vi "Load Becker-Hickl FLIM Data Block.vi"(4 "Compressed?":bool, 6 "Image Sizes":T1, 8 "Error In":errorcluster, 9 "Data Type":T3, 10 "Data Block Header":T2, 11 "File Path Control":path) -> (0 "Error Out":errorcluster, 2 "Data":sgl[][][](array[numeric]), 3 "File Path":path)   [LabVIEW 2021, in "Becker-Hickl Files.lvlib"]
uses:
  Becker-Hickl Files.lvlib
  Becker-Hickl Data Type.ctl
  Becker-Hickl Data Block Header.ctl
  Becker-Hickl FLIM Image Sizes.ctl
panel:
  out "Intensity Graph":sgl[][](graph)
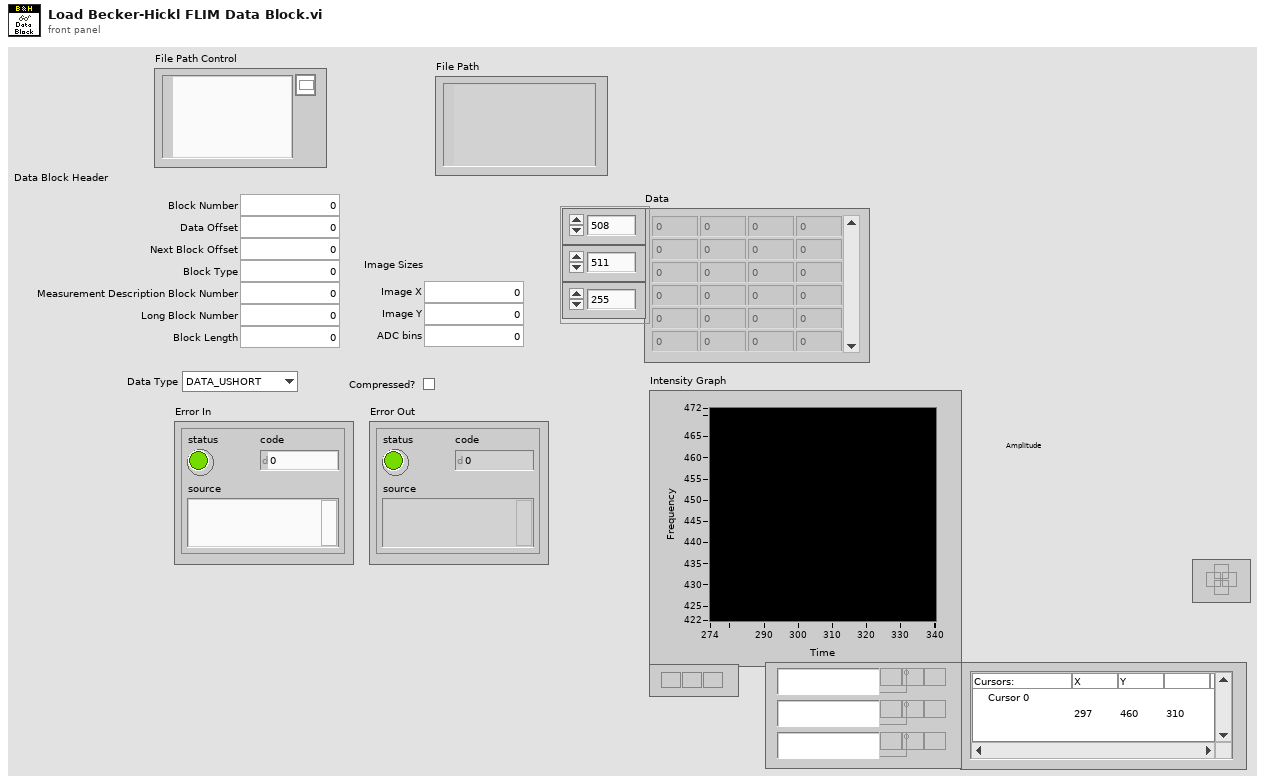
[diagram p1: front panel]
types:
  T1 = typedef "Becker-Hickl Files.lvlib/Becker-Hickl FLIM Image Sizes.ctl" = cluster{"Image X":i32, "Image Y":i32, "ADC bins":i32}
  T2 = typedef "Becker-Hickl Files.lvlib/Becker-Hickl Data Block Header.ctl" = cluster{"Block Number":u16, "Data Offset":u32, "Next Block Offset":u32, "Block Type":u16, "Measurement Description Block Number":u16, "Long Block Number":u32, "Block Length":u32}
  T3 = typedef "Becker-Hickl Files.lvlib/Becker-Hickl Data Type.ctl" = enum16{"DATA_USHORT", "DATA_ULONG", "DATA_DBL"}
  T4 = enum16{"big-endian, network order", "native, host order", "little-endian"}
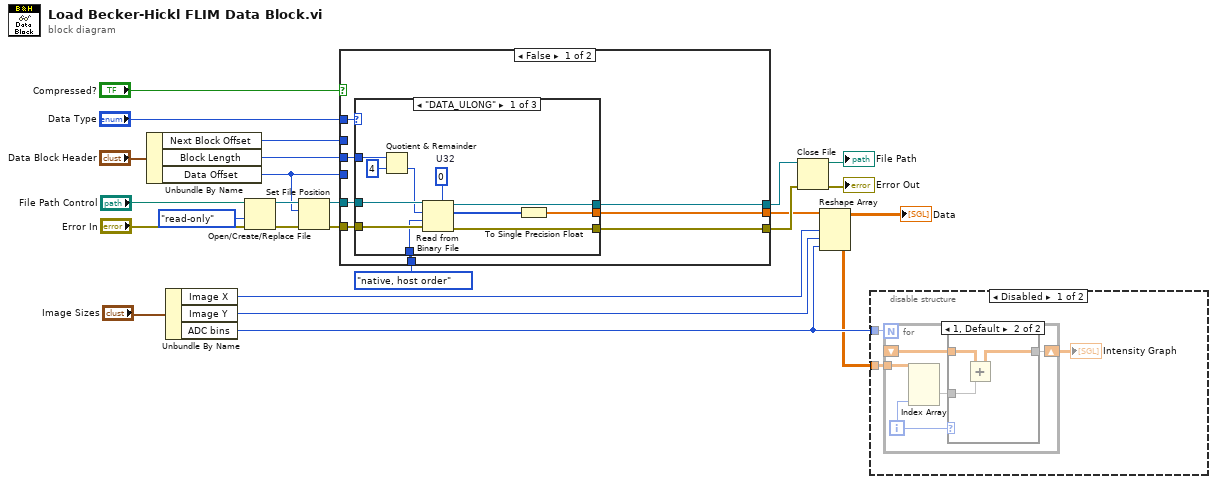
[diagram p0: block diagram]
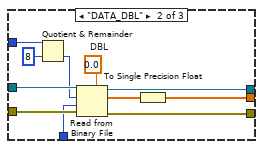
[diagram p4: hidden frame]
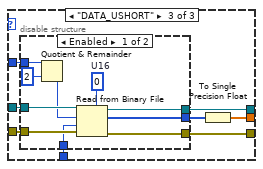
[diagram p5: hidden frame]
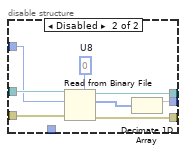
[diagram p6: hidden frame]
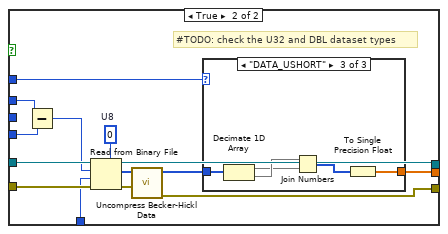
[diagram p7: hidden frame]
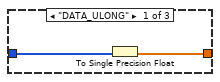
[diagram p8: hidden frame]
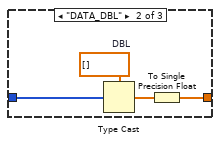
[diagram p9: hidden frame]
diagram:
  n1 = Unbundle By Name("Data Block Header") -> ("Next Block Offset"=w4:u32, "Block Length"=w15:u32, "Data Offset"=w3:u32)
  n2 = Unbundle By Name("Image Sizes") -> ("Image X"=w7:i32, "Image Y"=w6:i32, "ADC bins"=w2:i32)
  n3 = Open/Create/Replace File(file path (use dialog)="File Path Control", error in="Error In", access (0:read/write)=enum16{"read/write", "read-only", "write-only"}."read-only") -> (refnum out=w19:refnum<file>, error out=w20:errorcluster)  [unwired: 3 in, 1 out]
  n4 = Set File Position(offset (in bytes) (0)=w3, refnum=w19, error in=w20) -> (refnum out=w17:refnum<file>, error out=w16:errorcluster)  [unwired: 1 in]
  n5 = case shown="False" "Compressed?" {
    tunnel: "Data Type" -> [w32 w89]
    tunnel: w17 -> [w31 w93]
    tunnel: w16 -> [w30 w94]
    tunnel: w15 -> [w29 _]
    tunnel: [w28 w90] -> w14
    tunnel: [w27 w87] -> w13
    tunnel: [w26 w88] -> w10
    tunnel: T4."native, host order" ("byte order (0:big-endian, network order)") -> [w25 w81]
    tunnel: w4 -> [_ w92]
    tunnel: w3 -> [_ w91]
    frame False {
      n6 = case shown="\"DATA_ULONG\"" w32 {
        tunnel: w31 -> [w42 w53 w61]
        tunnel: w30 -> [w43 w54 w62]
        tunnel: w29 -> [w36 w47 w57]
        tunnel: [w40 w51 w60] -> w28
        tunnel: [w34 w45 w56] -> w26
        tunnel: [w38 w49 w58] -> w27
        tunnel: w25 -> [w33 w44 w55]
        frame "DATA_ULONG" {
          w41 = u32 0  # U32
          n7 = Quotient & Remainder(x=w36, y=u32 4) -> (floor(x/y)=w37:u32)  [unwired: 1 out]
          n8 = Read from Binary File(5:w41, 8:w43, 9:w33, 10:w37, 11:w42) -> (0:w38:errorcluster, 2:w39:u32[], 3:w40:refnum<file>)  [unwired: 1 in, 1 out]
          n9 = To Single Precision Float(number=w39) -> (single precision float=w34:sgl[])
        }
        frame "DATA_DBL" {
          w52 = 0.0  # DBL
          n10 = Quotient & Remainder(x=w47, y=u32 8) -> (floor(x/y)=w46:u32)  [unwired: 1 out]
          n11 = Read from Binary File(5:w52, 8:w54, 9:w44, 10:w46, 11:w53) -> (0:w49:errorcluster, 2:w50:dbl[], 3:w51:refnum<file>)  [unwired: 1 in, 1 out]
          n12 = To Single Precision Float(number=w50) -> (single precision float=w45:sgl[])
        }
        frame "DATA_USHORT" {
          n13 = disable-structure shown="Enabled" {
            disable-tunnel: w62 -> [w72 w80]
            disable-tunnel: w61 -> [w71 w79]
            disable-tunnel: [w69 w77] -> w60
            disable-tunnel: [w68 w73] -> w59
            disable-tunnel: [w67 w75] -> w58
            disable-tunnel: w57 -> [w65 w74]
            disable-tunnel: w55 -> [w63 _]
            frame Enabled {
              w70 = u16 0  # U16
              n14 = Quotient & Remainder(x=w65, y=u32 2) -> (floor(x/y)=w64:u32)  [unwired: 1 out]
              n15 = Read from Binary File(5:w70, 8:w72, 9:w63, 10:w64, 11:w71) -> (0:w67:errorcluster, 2:w68:u16[], 3:w69:refnum<file>)  [unwired: 1 in, 1 out]
            }
            frame Disabled {
              w78 = u8 0  # U8
              n16 = Read from Binary File(5:w78, 8:w80, 10:w74, 11:w79) -> (0:w75:errorcluster, 2:w76:u8[], 3:w77:refnum<file>)  [unwired: 2 in, 1 out]
              n17 = Decimate 1D Array(w76) -> (w73:u8[])  [unwired: 1 out]
            }
          }
          n18 = To Single Precision Float(number=w59) -> (single precision float=w56:sgl[])
        }
      }
    }
    frame True {
      w86 = u8 0  # U8
      # "#TODO: check the U32 and DBL dataset types"
      n19 = Subtract(x=w92, y=w91) -> (x-y=w85:u32)
      n20 = Read from Binary File(5:w86, 8:w94, 9:w81, 10:w85, 11:w93) -> (0:w84:errorcluster, 2:w83:u8[], 3:w90:refnum<file>)  [unwired: 1 in, 1 out]
      n21 = call "Uncompress Becker-Hickl Data.vi"("error in (no error)"=w84, "Compressed Data in"=w83) -> ("error out"=w87:errorcluster, "Uncompressed Data out"=w82:u8[])  [unwired: 6 in, 2 out]
      n22 = case shown="\"DATA_USHORT\"" w89 {
        tunnel: [w95 w97 w101] -> w88
        tunnel: w82 -> [w96 w99 w105]
        frame "DATA_ULONG" {
          n23 = To Single Precision Float(number=w96) -> (single precision float=w95:sgl[])
        }
        frame "DATA_DBL" {
          w100 = dbl[] []  # DBL
          n24 = Type Cast(type=w100, x=w99) -> (*(type *) &x=w98:dbl[])
          n25 = To Single Precision Float(number=w98) -> (single precision float=w97:sgl[])
        }
        frame "DATA_USHORT" {
          n26 = Decimate 1D Array(w105) -> (w103:u8[], w104:u8[])
          n27 = Join Numbers(hi=w104, lo=w103) -> ((hi.lo)=w102:u16[])
          n28 = To Single Precision Float(number=w102) -> (single precision float=w101:sgl[])
        }
      }
    }
  }
  n29 = Close File(refnum=w14, error in=w13) -> (path=→"File Path":path, error out=→"Error Out":errorcluster)
  n30 = Reshape Array(w10, w7, w6, w2) -> (w1:sgl[][][])
  "Data" <- w1
  n31 = disable-structure shown="Disabled" {
    disable-tunnel: w2 -> [w108 _]
    disable-tunnel: w1 -> [w107 _]
    frame Disabled {
      n32 = for {
        N: w108 -> [_]
        tunnel: w107 -> [w113]
        shift-right: [w111] -> w106
        shift-left: _ -> [w109]
        i -> [w112]
        n33 = Index Array(array=w113, index (dim 2)=w112) -> (element=w110:sgl[][])  [unwired: 2 in]
        n34 = case shown="1, Default" w112 {
          tunnel: [w114 w115] -> w111
          tunnel: w110 -> [w114 w116]
          tunnel: w109 -> [_ w117]
          frame 0 {
          }
          frame 1, Default {
            n35 = Add(x=w117, y=w116) -> (x+y=w115:sgl[][])
          }
        }
      }
      "Intensity Graph" <- w106
    }
    frame Enabled {
    }
  }
